vi "LaserMaster.vi"() -> ()   [LabVIEW 2014]
uses:
  <vilib>/Instr/_visa.llb/VISA Configure Serial Port (Instr).vi
  <vilib>/Utility/file.llb/Write To Spreadsheet File (string).vi
panel:
  out "Humidity Threshold":dbl
  in  "Power (mW) 2":dbl format="%#.0f"
  out "SavePath":path
  out "Start time":timestamp
  out "Step":dbl
  out "State next step":string
  in  "stop":bool
  out "Query backup List":string[][](array[string])=[["?L", " 0\r"], ["?K", " 0\r"], ["?F", " 0\r"], ["?FH", " 2\r"], ["?SHUTTER", " 0\r"], ["?UF", " 0\r"], ["?PHLDC", " 1\r"], ["?PZTMC", " 0\r"], ["?PZTXC", " 2.24\r"], ["?PZTYC", " 2.14\r"], ["?PHLDP", " 0\r"], ["?PZTMP", " 0\r"], ["?PZTXP", " 2.58\r"], ["?PXTYP", "  Query Error:?PXTYP\r"], ["?PTRK", "  Query Error:?PTRK\r"], ["?MDLK", " 0\r"], ["?PP", " 0.80\r"], ["?TS", " 0\r"], ["?SM", " 1\r"], ["?HM", " 1\r"], ["?VW", " 850\r"], ["?STPRPOS", " 2096\r"], ["?C", " 0.00\r"], ["?D1C", " 0.08\r"], ["?D2C", " -0.43\r"], ["?BT", " 20.07\r"], ["?D1T", " 24.20\r"], ["?D2T", " 24.20\r"], ["?VT", " 20.72\r"], ["?LBOT", " 148.45\r"], ["?ET", " 39.01\r"], ["?D1ST", " 24.20\r"], ["?D2ST", " 24.20\r"], ["?VST", " 30.00\r"], ["?LBOST", " 148.41\r"], ["?EST", " 39.00\r"], ["?D1TD", " 500.12\r"], ["?D2TD", " 464.53\r"], ["?VD", " 0.00\r"], ["?LBOD", " 5358.08\r"], ["?ED", " 2152.46\r"], ["?D1HST", " 21.35\r"], ["?D2HST", " 21.48\r"], ["?LBOH", " 1\r"], ["?LRS", " 2\r"], ["?D1SS", " 1\r"], ["?D2SS", " 1\r"], ["?VSS", " 0\r"], ["?LBOSS", " 1\r"], ["?ESS", " 1\r"], ["?D1H", "  351.54\r"], ["?D2H", "  351.52\r"], ["?HH", " 37\r"], ["?D1V", " 0.19\r"], ["?D2V", " 0.18\r"], ["?SV", " 8.26,8.26,9.57\r"], ["?MB", "  Query Error:?MB\r"], ["?PI", " 2BC\r"], ["?BV", " 13.24\r"], ["?AMDLK", " 1\r"], ["?PZTS", "  Query Error:?PZTS\r"], ["?TMAX", " 1080\r"], ["?TMIN", " 680\r"], ["?ALIGN", " 0\r"], ["?ALIGNP", " 250\r"], ["?ALIGNW", " 730\r"], ["?LFP", " 0\r"], ["?PZTXCM", " 8.11\r"], ["?PZTXCP", " -10.30\r"], ["?PZTXPM", " 8.11\r"], ["?PZTXPP", " 3.06\r"], ["?PZTYCM", " 8.11\r"], ["?PZTYCP", " -14.28\r"], ["?PZTYPM", " 8.11\r"], ["?PZTYPP", " 11.74\r"], ["?RH", " 0\r"], ["?SN", " 9571\r"], ["?ST", " Standby\r"], ["?GDDCURVE", " 0\r"], ["?GDD", " 0\r"], ["?GDDCURVEN", " ZERO\r"], ["?CURVEN", " OUT OF RANGE\r"], ["?COMP", " 1\r"], ["?HMCOMP", " 1\r"], ["?GDDMAX", " 17333\r"], ["?GDDMIN", "0"]]
  out "Laser Info":i32
  out "Shutter off time":dbl
  out "Quiting":dbl
  out "Backuper state":string
  in  "Tab Control":T1(tab)
  in  "Auto":bool
  out "Baseplate Temp (C)":dbl(slide) scale=20.0..40.0
  in  "Dither hold":bool
  in  "Shutter":bool
  in  "Lock":bool
  out "Laser Status":bool
  out "Power (mW)":dbl(knob) scale=0.0..5000.0
  out "Walking":bool
  out "Sleeping":bool
  out "ModeLocked":bool
  out "Backing up":bool
  in  "Wavelength":dbl
  in  "GDD":dbl
  in  "Align":bool
  in  "QUIT":bool
  out "Max":string
  in  "Dither auto":dbl=120.0
  in  "Dither timer":dbl=5.0
  out "Faults":string
  in  "Home motor":bool
  in  "Optimize":bool
  in  "WV Walk":bool
  in  "Auto-Standby\nTime (min)":dbl=120.0
  in  "Sleep":bool
  in  "Backup":bool
  in  "Auto-Backup \nIdle Time (min)":dbl=30.0
  out "Operating Status":string
  out "Tunning Status":i32
  out "Idle Time":dbl format="%.1f"
  out "Laser On Time":dbl format="%#.1f"
  in  "Laser Control":bool
  in  "Command Line":string
  out "Laser Response":string
  in  "Refresh":bool
  out "Query List":string[][](array[string])
  out "queue #":i32
  # "LASER"
  # "LASER fine-tune"
  # "BACKUP"
  # "Timers"
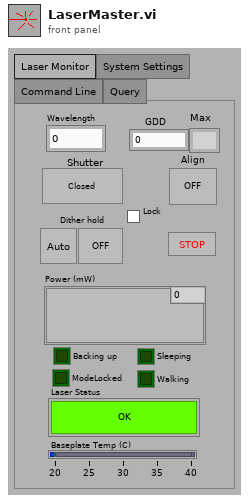
[diagram p1: front panel]
types:
  T1 = enum32{"Laser Monitor", "System Settings", "Command Line", "Query"}
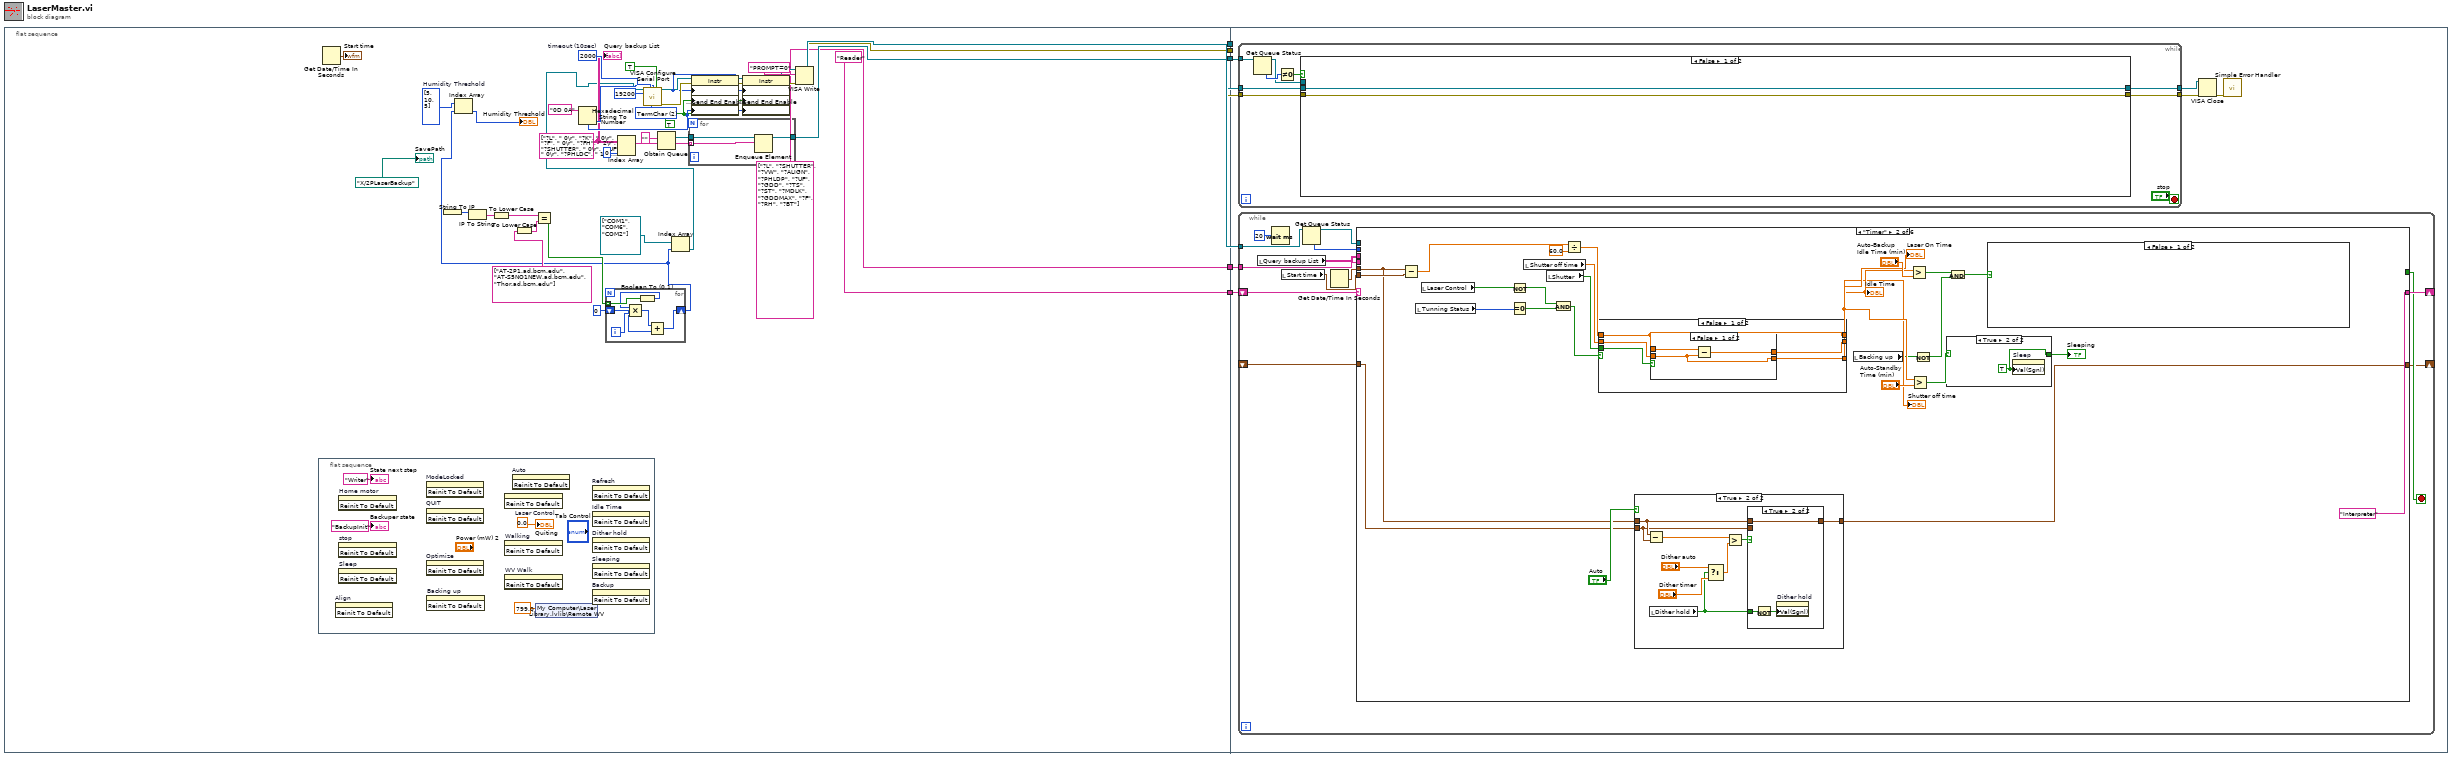
[diagram p0: block diagram]
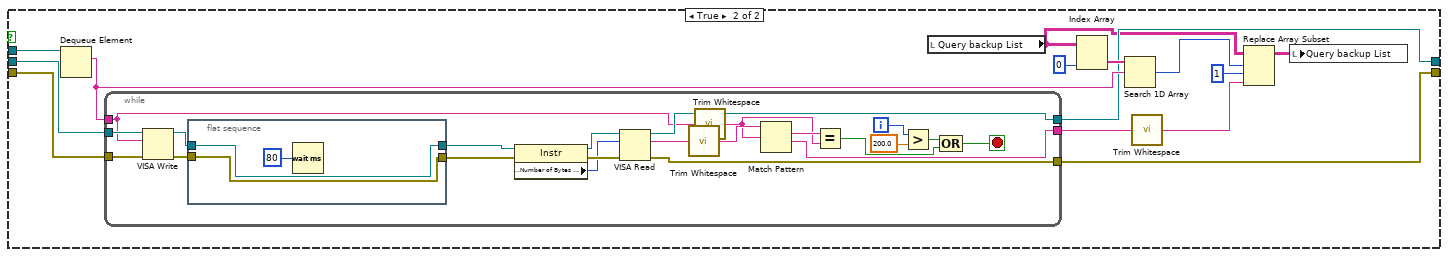
[diagram p2: hidden frame]
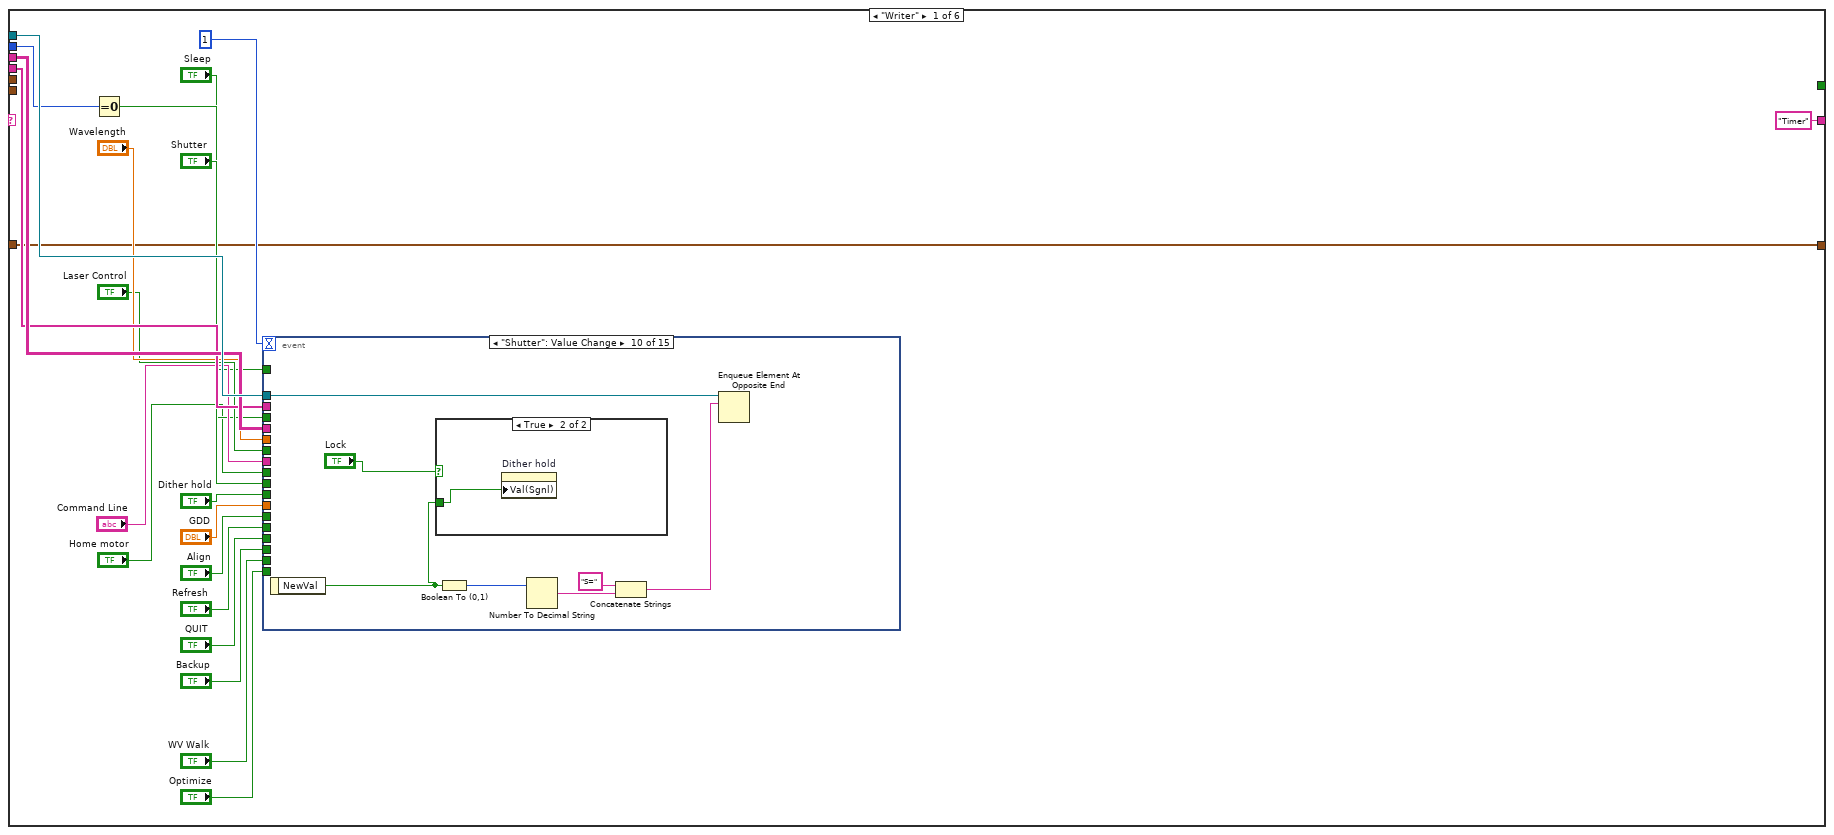
[diagram p3: hidden frame]
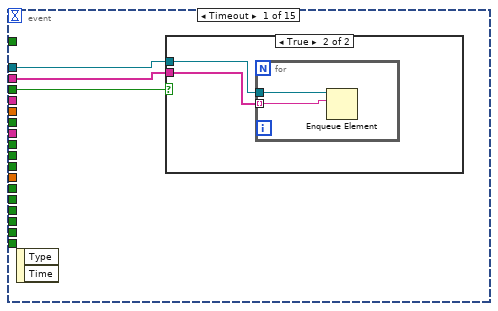
[diagram p4: hidden frame]
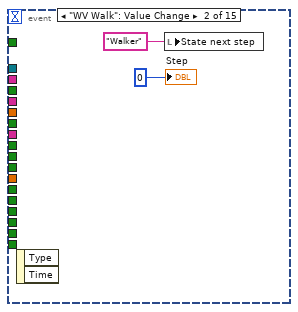
[diagram p6: hidden frame]
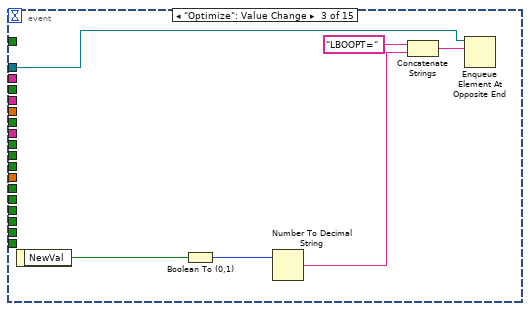
[diagram p7: hidden frame]
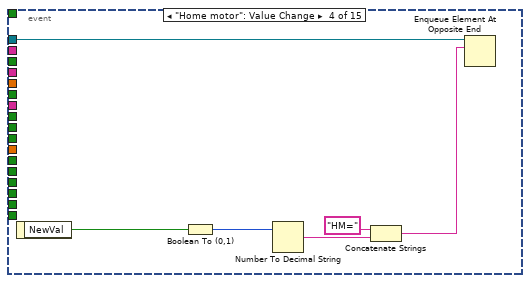
[diagram p8: hidden frame]
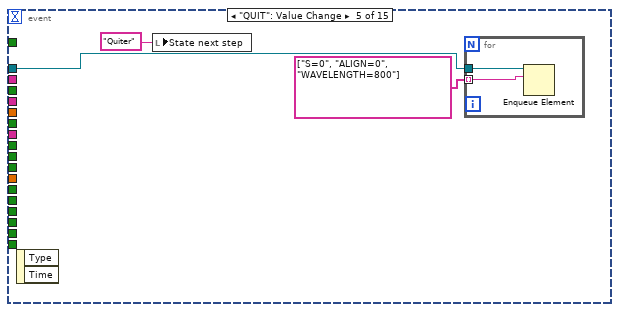
[diagram p9: hidden frame]
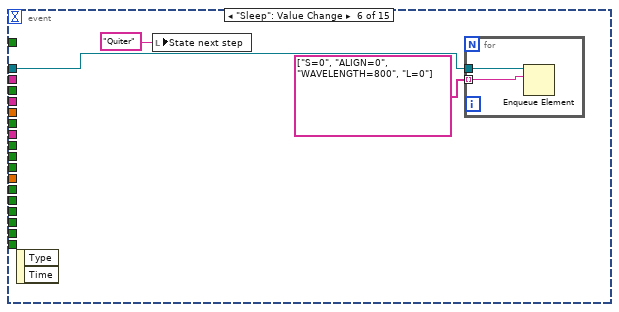
[diagram p10: hidden frame]
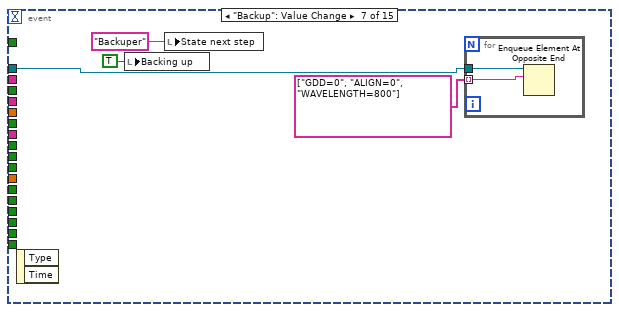
[diagram p11: hidden frame]
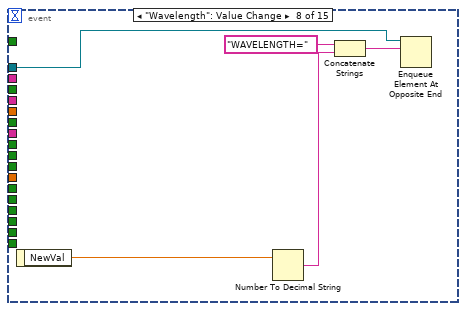
[diagram p12: hidden frame]
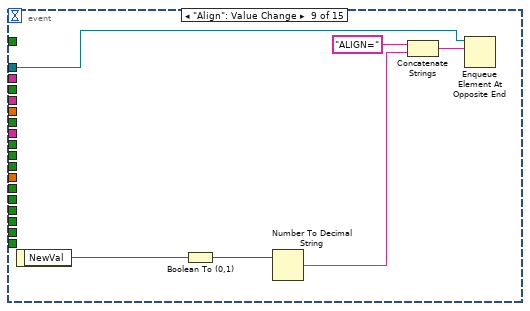
[diagram p13: hidden frame]
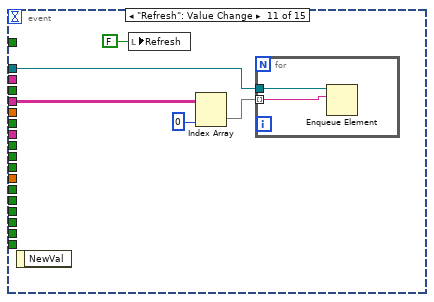
[diagram p15: hidden frame]
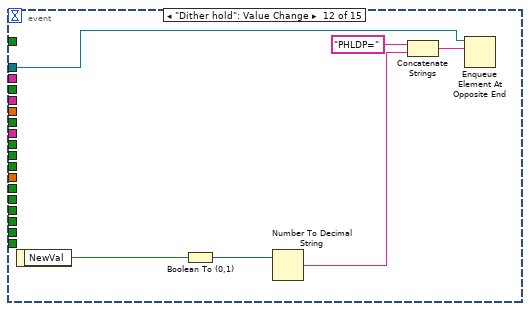
[diagram p16: hidden frame]
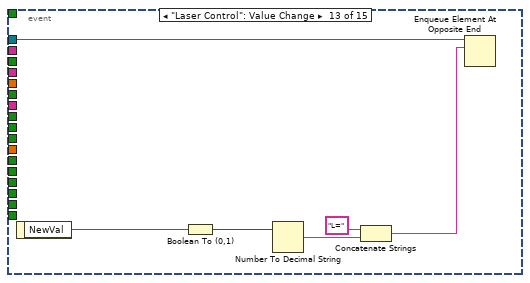
[diagram p17: hidden frame]
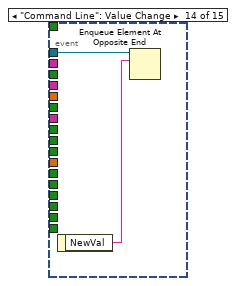
[diagram p18: hidden frame]
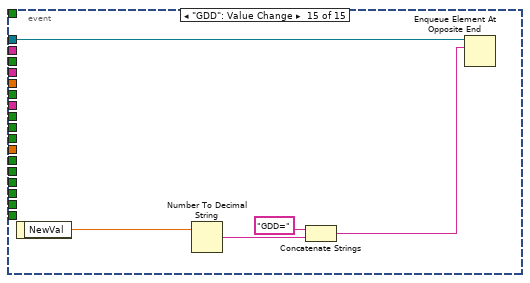
[diagram p19: hidden frame]
diagram:
  n1 = flat-sequence {
    tunnel: [w32] -> w5
    tunnel: [w31] -> w4
    tunnel: [w22] -> w3
    tunnel: [string[] ["?L", "?SHUTTER", "?VW", "?ALIGN", "?PHLDP", "?UF", "?GDD", "?TS", "?ST", "?MDLK", "?GDDMAX", "?F", "?RH", "?BT"]] -> w2
    tunnel: ["Reader"] -> w1
    tunnel: w5 -> [w60]
    tunnel: w4 -> [w57]
    tunnel: w3 -> [w61]
    tunnel: w2 -> [w63]
    tunnel: w1 -> [w62]
    frame #0 {
      w8 = i32[] [5, 10, 5]  # Humidity Threshold
      w21 = string[][] [["?L", " 0\r"], ["?K", " 0\r"], ["?F", " 0\r"], ["?FH", " 2\r"], ["?SHUTTER", " 0\r"], ["?UF", " 0\r"], ["?PHLDC", " 1\r"], ["?PZTMC", " 0\r"], ["?PZTXC", " 2.24\r"], ["?PZTYC", " 2.14\r"], ["?PHLDP", " 0\r"], ["?PZTMP", " 0\r"], ["?PZTXP", " 2.58\r"], ["?PXTYP", "  Query Error:?PXTYP\r"], ["?PTRK", "  Query Error:?PTRK\r"], ["?MDLK", " 0\r"], ["?PP", " 0.80\r"], ["?TS", " 0\r"], ["?SM", " 1\r"], ["?HM", " 1\r"], ["?VW", " 850\r"], ["?STPRPOS", " 2096\r"], ["?C", " 0.00\r"], ["?D1C", " 0.08\r"], ["?D2C", " -0.43\r"], ["?BT", " 20.07\r"], ["?D1T", " 24.20\r"], ["?D2T", " 24.20\r"], ["?VT", " 20.72\r"], ["?LBOT", " 148.45\r"], ["?ET", " 39.01\r"], ["?D1ST", " 24.20\r"], ["?D2ST", " 24.20\r"], ["?VST", " 30.00\r"], ["?LBOST", " 148.41\r"], ["?EST", " 39.00\r"], ["?D1TD", " 500.12\r"], ["?D2TD", " 464.53\r"], ["?VD", " 0.00\r"], ["?LBOD", " 5358.08\r"], ["?ED", " 2152.46\r"], ["?D1HST", " 21.35\r"], ["?D2HST", " 21.48\r"], ["?LBOH", " 1\r"], ["?LRS", " 2\r"], ["?D1SS", " 1\r"], ["?D2SS", " 1\r"], ["?VSS", " 0\r"], ["?LBOSS", " 1\r"], ["?ESS", " 1\r"], ["?D1H", "  351.54\r"], ["?D2H", "  351.52\r"], ["?HH", " 37\r"], ["?D1V", " 0.19\r"], ["?D2V", " 0.18\r"], ["?SV", " 8.26,8.26,9.57\r"], ["?MB", "  Query Error:?MB\r"], ["?PI", " 2BC\r"], ["?BV", " 13.24\r"], ["?AMDLK", " 1\r"], ["?PZTS", "  Query Error:?PZTS\r"], ["?TMAX", " 1080\r"], ["?TMIN", " 680\r"], ["?ALIGN", " 0\r"], ["?ALIGNP", " 250\r"], ["?ALIGNW", " 730\r"], ["?LFP", " 0\r"], ["?PZTXCM", " 8.11\r"], ["?PZTXCP", " -10.30\r"], ["?PZTXPM", " 8.11\r"], ["?PZTXPP", " 3.06\r"], ["?PZTYCM", " 8.11\r"], ["?PZTYCP", " -14.28\r"], ["?PZTYPM", " 8.11\r"], ["?PZTYPP", " 11.74\r"], ["?RH", " 0\r"], ["?SN", " 9571\r"], ["?ST", " Standby\r"], ["?GDDCURVE", " 0\r"], ["?GDD", " 0\r"], ["?GDDCURVEN", " ZERO\r"], ["?CURVEN", " OUT OF RANGE\r"], ["?COMP", " 1\r"], ["?HMCOMP", " 1\r"], ["?GDDMAX", " 17333\r"], ["?GDDMIN", "0"]] ("Query backup List")
      w35 = TRUE ("Message Based Settings:Send End Enable")
      w36 = u16 2 items=["None", "LastBit", "TermChar", "Break"] ("Serial Settings:Serial End Mode for Writes")
      w43 = u32 2000  # timeout (10sec)
      n2 = flat-sequence {
        frame #0 {
          n3 = invoke on="Align" class="Bool (strict)" method="Reinit To Default"() -> ()  [unwired: 3 in, 3 out]
          n4 = invoke on="Home motor" class="Bool" method="Reinit To Default"() -> ()  [unwired: 3 in, 3 out]
          n5 = invoke on="stop" class="Bool (strict)" method="Reinit To Default"() -> ()  [unwired: 3 in, 3 out]
          n6 = invoke on="Sleep" class="Bool (strict)" method="Reinit To Default"() -> ()  [unwired: 3 in, 3 out]
          n7 = invoke on="ModeLocked" class="Bool (strict)" method="Reinit To Default"() -> ()  [unwired: 3 in, 3 out]
          n8 = invoke on="QUIT" class="Bool (strict)" method="Reinit To Default"() -> ()  [unwired: 3 in, 3 out]
          n9 = invoke on="Optimize" class="Bool" method="Reinit To Default"() -> ()  [unwired: 3 in, 3 out]
          n10 = invoke on="Backing up" class="Bool (strict)" method="Reinit To Default"() -> ()  [unwired: 3 in, 3 out]
          n11 = invoke on="Laser Control" class="Bool (strict)" method="Reinit To Default"() -> ()  [unwired: 3 in, 3 out]
          n12 = invoke on="Walking" class="Bool (strict)" method="Reinit To Default"() -> ()  [unwired: 3 in, 3 out]
          n13 = invoke on="WV Walk" class="Bool (strict)" method="Reinit To Default"() -> ()  [unwired: 3 in, 3 out]
          n14 = invoke on="Auto" class="Bool (strict)" method="Reinit To Default"() -> ()  [unwired: 3 in, 3 out]
          n15 = shared-variable "My Computer\\Laser Library.lvlib\\Remote WV"(799.0 ("Remote WV")) -> ()  [unwired: 1 in, 1 out]
          n16 = invoke on="Refresh" class="Bool (strict)" method="Reinit To Default"() -> ()  [unwired: 3 in, 3 out]
          n17 = invoke on="Idle Time" class="DigNum (strict)" method="Reinit To Default"() -> ()  [unwired: 3 in, 3 out]
          n18 = invoke on="Dither hold" class="Bool (strict)" method="Reinit To Default"() -> ()  [unwired: 3 in, 3 out]
          n19 = invoke on="Sleeping" class="Bool (strict)" method="Reinit To Default"() -> ()  [unwired: 3 in, 3 out]
          n20 = invoke on="Backup" class="Bool (strict)" method="Reinit To Default"() -> ()  [unwired: 3 in, 3 out]
          "Backuper state" <- "BackupInit"
          "Quiting" <- 0.0 ("Quiting")
          "State next step" <- "Writer"
        }
      }
      n21 = Get Date/Time In Seconds() -> (seconds since 1Jan1904=→"Start time":timestamp)
      n22 = String To IP() -> (0:w17:u32)  [unwired: 1 in]
      n23 = IP To String(2:w17) -> (0:w14:string)  [unwired: 1 in]
      n24 = To Lower Case(string=w14) -> (all lower case string=w16:string)
      n25 = To Lower Case(string=string[] ["AT-2P1.ad.bcm.edu", "AT-S5NO1NEW.ad.bcm.edu", "Thor.ad.bcm.edu"]) -> (all lower case string=w15:string[])
      n26 = Equal?(x=w16, y=w15) -> (x = y?=w11:bool[])
      n27 = Hexadecimal String To Number(string="0D 0A") -> (number=w34:u32)  [unwired: 2 in, 1 out]
      n28 = for {
        tunnel: w11 -> [w48] mode=indexing
        shift-right: [w44] -> w7
        shift-left: 0 -> [w45]
        i -> [w49]
        n29 = Boolean To (0,1)(Boolean=w48) -> (0, 1=w47:i16)
        n30 = Multiply(x=w47, y=w49) -> (x*y=w46:i32)
        n31 = Add(x=w46, y=w45) -> (x+y=w44:i32)
      }
      n32 = Index Array(array=w8, index=w7) -> (element=→"Humidity Threshold":i32)
      n33 = Index Array(array=w21, index (col)=0 ("disabled index (col)")) -> (element=w24:string[])  [unwired: 1 in]
      n34 = Obtain Queue(element data type="") -> (queue out=w26:refnum<queue>)  [unwired: 4 in, 2 out]
      n35 = Index Array(array=refnum<visa-resource-name>[] ["COM1", "COM6", "COM2"], index=w7) -> (element=w9:refnum<visa-resource-name>)
      n36 = call-poly "VISA Configure Serial Port"("VISA resource name"=w9, "timeout (10sec)"=w43, "termination char\n(0xA = '\\n' = LF)"=w34, "Enable Termination\nChar (T)"=TRUE ("Enable Termination\nChar (T)"), "baud rate (9600)"=u32 19200) -> ("VISA resource name out"=w40:refnum<visa-resource-name>, "error out"=w39:errorcluster)  [unwired: 5 in, 4 out]
      n37 = for {
        tunnel: w26 -> [w56]
        tunnel: w24 -> [w55] mode=indexing
        tunnel: [w54] -> w22
        n38 = Enqueue Element(queue=w56, element=w55) -> (queue out=w54:refnum<queue>)  [unwired: 2 in, 2 out]
      }
      n39 = property class="Instr"(reference=w40, error in=w39, "Serial Settings:End Mode for Writes"=w36, "Message Based Settings:Send End Enable"=w35, "Message Based Settings:Termination Character"=w34) -> (reference out=w38:refnum<visa-resource-name>, error out=w37:errorcluster)
      n40 = property class="Instr"(reference=w38, error in=w37, "Serial Settings:End Mode for Writes"=w36, "Message Based Settings:Send End Enable"=w35, "Message Based Settings:Termination Character"=w34) -> (reference out=w29:refnum<visa-resource-name>, error out=w28:errorcluster)
      n41 = VISA Write(VISA resource name=w29, write buffer="PROMPT=0", error in (no error)=w28) -> (VISA resource name out=w32:refnum<visa-resource-name>, error out=w31:errorcluster)  [unwired: 1 out]
      "Query backup List" <- w21
      "SavePath" <- path "X:/2PLaserBackup"
    }
    frame #1 {
      n42 = while {
        tunnel: w61 -> [w68]
        tunnel: w60 -> [w73]
        tunnel: [w72] -> w59
        tunnel: [w71] -> w58
        tunnel: w57 -> [w70]
        stop <- "stop" stop-if-true
        n43 = Get Queue Status(queue=w68) -> (queue out=w65:refnum<queue>, # elements in queue=w67:i32)  [unwired: 2 in, 6 out]
        n44 = Not Equal To 0?(x=w67) -> (x != 0?=w66:bool)
        n45 = case shown="False" w66 {
          tunnel: w65 -> [_ w82]
          tunnel: w73 -> [w75 w81]
          tunnel: [w75 w80] -> w72
          tunnel: [w74 w79] -> w71
          tunnel: w70 -> [w74 w78]
          frame False {
          }
          frame True {
            n46 = Dequeue Element(queue=w82) -> (element=w84:string)  [unwired: 2 in, 3 out]
            n47 = while {
              tunnel: w81 -> [w111]
              tunnel: w78 -> [w110]
              tunnel: [w109] -> w80
              tunnel: [w108] -> w79
              tunnel: w84 -> [w96]
              tunnel: [w104] -> w85
              i -> [w94]
              stop <- w91 stop-if-true
              n48 = VISA Write(VISA resource name=w111, write buffer=w96, error in (no error)=w110) -> (VISA resource name out=w102:refnum<visa-resource-name>, error out=w99:errorcluster)  [unwired: 1 out]
              n49 = flat-sequence {
                tunnel: [w114] -> w101
                tunnel: w102 -> [w114]
                tunnel: w99 -> [w113]
                tunnel: [w113] -> w100
                frame #0 {
                  n50 = Wait (ms)(milliseconds to wait=u32 80) -> ()  [unwired: 1 out]
                }
              }
              n51 = property class="Instr"(reference=w101, error in=w100) -> (reference out=w107:refnum<visa-resource-name>, error out=w106:errorcluster, "Serial Settings:Number of Bytes at Serial Port"=w105:u32)
              n52 = VISA Read(VISA resource name=w107, byte count=w105, error in (no error)=w106) -> (VISA resource name out=w109:refnum<visa-resource-name>, read buffer=w98:string, error out=w108:errorcluster)  [unwired: 1 out]
              n53 = call <vilib>:"Trim Whitespace.vi"("string"=w98) -> ("trimmed string"=w97:string)  [unwired: 1 in]
              n54 = call <vilib>:"Trim Whitespace.vi"("string"=w96) -> ("trimmed string"=w90:string)  [unwired: 1 in]
              n55 = Match Pattern(string=w97, regular expression=w90) -> (match substring=w103:string, after substring=w104:string)  [unwired: 1 in, 2 out]
              n56 = Equal?(x=w103, y=w90) -> (x = y?=w92:bool)
              n57 = Greater?(x=w94, y=200.0) -> (0:w93:bool)
              n58 = Compound Arithmetic op=OR(w93, w92) -> (w91:bool)
            }
            n59 = local read "Query backup List"() -> (w77:string[][])
            n60 = Index Array(array=w77, index (col)=0 ("index (row)")) -> (element=w88:string[])  [unwired: 1 in]
            n61 = Search 1D Array(1D array=w88, element=w84) -> (index of element=w86:i32)  [unwired: 1 in]
            n62 = call <vilib>:"Trim Whitespace.vi"("string"=w85) -> ("trimmed string"=w83:string)  [unwired: 1 in]
            n63 = Replace Array Subset(array=w77, new element=w83, index (row)=w86, index (col)=1 ("disabled index (col)")) -> (w76:string[][])
            n64 = local write "Query backup List"(w76) -> ()
          }
        }
      }
      n65 = while {
        tunnel: w61 -> [w124]
        tunnel: w63 -> [w125]
        shift-right: [w126] -> _
        shift-left: w62 -> [w127]
        shift-right: [w116] -> _
        shift-left: _ -> [w115]
        stop <- w121 stop-if-true
        n66 = local read "Query backup List"() -> (w123:string[][])
        n67 = Wait (ms)(milliseconds to wait=u32 20) -> ()  [unwired: 1 out]
        n68 = local read "Start time"() -> (w117:timestamp)
        n69 = Get Queue Status(queue=w124) -> (queue out=w120:refnum<queue>, # elements in queue=w119:i32)  [unwired: 2 in, 6 out]
        n70 = Get Date/Time In Seconds() -> (seconds since 1Jan1904=w118:timestamp)
        n71 = case shown="\"Timer\"" w127 {
          tunnel: w120 -> [w149 _ _ _ _ _]
          tunnel: w123 -> [w148 _ w302 _ w457 _]
          tunnel: w125 -> [w147 _ w303 _ _ _]
          tunnel: ["Timer" "Interpreter" w301 "Writer" "Writer" w483] -> w126
          tunnel: w119 -> [w146 _ w300 _ _ w485]
          tunnel: [_ _ _ _ _ w482] -> w121
          tunnel: w118 -> [_ w233 _ _ _ _]
          tunnel: w117 -> [_ w237 _ _ _ _]
          tunnel: [w128 w234 w299 w439 w454 w481] -> w116
          tunnel: w115 -> [w128 w232 w299 w439 w454 w481]
          frame "Writer" {
            n72 = Equal To 0?(x=w146) -> (x = 0?=w134:bool)
            n73 = event shown="[9] \"Shutter\": Value Change" {
              selector: _ -> [_ _ _ _ _ _ _ _ _ _ _ _ _ _ _]
              dyn-events: _ -> [_ _ _ _ _ _ _ _ _ _ _ _ _ _ _]
              timeout: 1 -> [_ _ _ _ _ _ _ _ _ _ _ _ _ _ _]
              tunnel: w149 -> [w152 _ w159 w166 w172 w176 w183 w188 w193 w200 w207 w214 w219 w226 w228]
              tunnel: "Shutter" -> [_ _ _ _ _ _ _ _ _ _ _ _ _ _ _]
              tunnel: "Dither hold" -> [_ _ _ _ _ _ _ _ _ _ _ _ _ _ _]
              tunnel: "GDD" -> [_ _ _ _ _ _ _ _ _ _ _ _ _ _ _]
              tunnel: "Align" -> [_ _ _ _ _ _ _ _ _ _ _ _ _ _ _]
              tunnel: "Wavelength" -> [_ _ _ _ _ _ _ _ _ _ _ _ _ _ _]
              tunnel: "Laser Control" -> [_ _ _ _ _ _ _ _ _ _ _ _ _ _ _]
              tunnel: "Command Line" -> [_ _ _ _ _ _ _ _ _ _ _ _ _ _ _]
              tunnel: w148 -> [_ _ _ _ _ _ _ _ _ _ w206 _ _ _ _]
              tunnel: "Refresh" -> [_ _ _ _ _ _ _ _ _ _ _ _ _ _ _]
              tunnel: w147 -> [w151 _ _ _ _ _ _ _ _ _ _ _ _ _ _]
              tunnel: "QUIT" -> [_ _ _ _ _ _ _ _ _ _ _ _ _ _ _]
              tunnel: "Backup" -> [_ _ _ _ _ _ _ _ _ _ _ _ _ _ _]
              tunnel: w134 -> [w150 _ _ _ _ _ _ _ _ _ _ _ _ _ _]
              tunnel: "WV Walk" -> [_ _ _ _ _ _ _ _ _ _ _ _ _ _ _]
              tunnel: "Optimize" -> [_ _ _ _ _ _ _ _ _ _ _ _ _ _ _]
              tunnel: "Home motor" -> [_ _ _ _ _ _ _ _ _ _ _ _ _ _ _]
              tunnel: "Sleep" -> [_ _ _ _ _ _ _ _ _ _ _ _ _ _ _]
              event Timeout {
                n74 = event-data() -> ()  [unwired: 1 in, 2 out]
                n75 = case shown="True" w150 {
                  tunnel: w152 -> [_ w154]
                  tunnel: w151 -> [_ w153]
                  frame False {
                  }
                  frame True {
                    n76 = for {
                      tunnel: w154 -> [w156]
                      tunnel: w153 -> [w155] mode=indexing
                      n77 = Enqueue Element(queue=w156, element=w155) -> ()  [unwired: 2 in, 3 out]
                    }
                  }
                }
              }
              event "WV Walk": Value Change {
                n78 = event-data() -> ()  [unwired: 1 in, 2 out]
                n79 = local write "State next step"("Walker") -> ()
                "Step" <- 0
              }
              event "Optimize": Value Change {
                n80 = event-data() -> ("NewVal"=w160:bool)  [unwired: 1 in]
                n81 = Boolean To (0,1)(Boolean=w160) -> (0, 1=w163:i16)
                n82 = Number To Decimal String(number=w163) -> (decimal integer string=w164:string)  [unwired: 1 in]
                n83 = Concatenate Strings("LBOOPT=", w164) -> (w161:string)
                n84 = Enqueue Element At Opposite End(queue=w159, element=w161) -> ()  [unwired: 2 in, 3 out]
              }
              event "Home motor": Value Change {
                n85 = event-data() -> ("NewVal"=w165:bool)  [unwired: 1 in]
                n86 = Boolean To (0,1)(Boolean=w165) -> (0, 1=w169:i16)
                n87 = Number To Decimal String(number=w169) -> (decimal integer string=w170:string)  [unwired: 1 in]
                n88 = Concatenate Strings("HM=", w170) -> (w167:string)
                n89 = Enqueue Element At Opposite End(queue=w166, element=w167) -> ()  [unwired: 2 in, 3 out]
              }
              event "QUIT": Value Change {
                n90 = event-data() -> ()  [unwired: 1 in, 2 out]
                n91 = local write "State next step"("Quiter") -> ()
                n92 = for {
                  tunnel: w172 -> [w175]
                  tunnel: string[] ["S=0", "ALIGN=0", "WAVELENGTH=800"] -> [w174] mode=indexing
                  n93 = Enqueue Element(queue=w175, element=w174) -> ()  [unwired: 2 in, 3 out]
                }
              }
              event "Sleep": Value Change {
                n94 = event-data() -> ()  [unwired: 1 in, 2 out]
                n95 = local write "State next step"("Quiter") -> ()
                n96 = for {
                  tunnel: w176 -> [w180]
                  tunnel: string[] ["S=0", "ALIGN=0", "WAVELENGTH=800", "L=0"] -> [w179] mode=indexing
                  n97 = Enqueue Element(queue=w180, element=w179) -> ()  [unwired: 2 in, 3 out]
                }
              }
              event "Backup": Value Change {
                n98 = event-data() -> ()  [unwired: 1 in, 2 out]
                n99 = local write "Backing up"(TRUE ("Backing up ...")) -> ()
                n100 = local write "State next step"("Backuper") -> ()
                n101 = for {
                  tunnel: string[] ["GDD=0", "ALIGN=0", "WAVELENGTH=800"] -> [w186] mode=indexing
                  tunnel: w183 -> [w185]
                  n102 = Enqueue Element At Opposite End(queue=w185, element=w186) -> ()  [unwired: 2 in, 3 out]
                }
              }
              event "Wavelength": Value Change {
                n103 = event-data() -> ("NewVal"=w187:dbl)  [unwired: 1 in]
                n104 = Number To Decimal String(number=w187) -> (decimal integer string=w190:string)  [unwired: 1 in]
                n105 = Concatenate Strings("WAVELENGTH=", w190) -> (w191:string)
                n106 = Enqueue Element At Opposite End(queue=w188, element=w191) -> ()  [unwired: 2 in, 3 out]
              }
              event "Align": Value Change {
                n107 = event-data() -> ("NewVal"=w192:bool)  [unwired: 1 in]
                n108 = Boolean To (0,1)(Boolean=w192) -> (0, 1=w196:i16)
                n109 = Number To Decimal String(number=w196) -> (decimal integer string=w197:string)  [unwired: 1 in]
                n110 = Concatenate Strings("ALIGN=", w197) -> (w194:string)
                n111 = Enqueue Element At Opposite End(queue=w193, element=w194) -> ()  [unwired: 2 in, 3 out]
              }
              event "Shutter": Value Change {
                n112 = event-data() -> ("NewVal"=w198:bool)  [unwired: 1 in]
                n113 = case shown="True" "Lock" {
                  tunnel: w198 -> [_ w205]
                  frame False {
                  }
                  frame True {
                    n114 = property on="Dither hold" class="Bool (strict)"("Val(Sgnl)"=w205) -> ()  [unwired: 2 in, 2 out]
                  }
                }
                n115 = Boolean To (0,1)(Boolean=w198) -> (0, 1=w203:i16)
                n116 = Number To Decimal String(number=w203) -> (decimal integer string=w204:string)  [unwired: 1 in]
                n117 = Concatenate Strings("S=", w204) -> (w201:string)
                n118 = Enqueue Element At Opposite End(queue=w200, element=w201) -> ()  [unwired: 2 in, 3 out]
              }
              event "Refresh": Value Change {
                n119 = event-data() -> ()  [unwired: 1 in, 1 out]
                n120 = local write "Refresh"(FALSE ("Backup")) -> ()
                n121 = Index Array(array=w206, index (col)=0 ("disabled index (col)")) -> (element=w209:string[])  [unwired: 1 in]
                n122 = for {
                  tunnel: w207 -> [w212]
                  tunnel: w209 -> [w211] mode=indexing
                  n123 = Enqueue Element(queue=w212, element=w211) -> ()  [unwired: 2 in, 3 out]
                }
              }
              event "Dither hold": Value Change {
                n124 = event-data() -> ("NewVal"=w213:bool)  [unwired: 1 in]
                n125 = Boolean To (0,1)(Boolean=w213) -> (0, 1=w217:i16)
                n126 = Number To Decimal String(number=w217) -> (decimal integer string=w218:string)  [unwired: 1 in]
                n127 = Concatenate Strings("PHLDP=", w218) -> (w215:string)
                n128 = Enqueue Element At Opposite End(queue=w214, element=w215) -> ()  [unwired: 2 in, 3 out]
              }
              event "Laser Control": Value Change {
                n129 = event-data() -> ("NewVal"=w220:bool)  [unwired: 1 in]
                n130 = Boolean To (0,1)(Boolean=w220) -> (0, 1=w223:i16)
                n131 = Number To Decimal String(number=w223) -> (decimal integer string=w224:string)  [unwired: 1 in]
                n132 = Concatenate Strings("L=", w224) -> (w221:string)
                n133 = Enqueue Element At Opposite End(queue=w219, element=w221) -> ()  [unwired: 2 in, 3 out]
              }
              event "Command Line": Value Change {
                n134 = event-data() -> ("NewVal"=w225:string)  [unwired: 1 in]
                n135 = Enqueue Element At Opposite End(queue=w226, element=w225) -> ()  [unwired: 2 in, 3 out]
              }
              event "GDD": Value Change {
                n136 = event-data() -> ("NewVal"=w227:dbl)  [unwired: 1 in]
                n137 = Number To Decimal String(number=w227) -> (decimal integer string=w230:string)  [unwired: 1 in]
                n138 = Concatenate Strings("GDD=", w230) -> (w231:string)
                n139 = Enqueue Element At Opposite End(queue=w228, element=w231) -> ()  [unwired: 2 in, 3 out]
              }
            }
          }
          frame "Timer" {
            n140 = Subtract(x=w233, y=w237) -> (x-y=w240:dbl)
            n141 = local read "Tunning Status"() -> (w257:i32)
            n142 = local read "Laser Control"() -> (w256:bool)
            n143 = Not(x=w256) -> (.not. x?=w252:bool)
            n144 = Equal To 0?(x=w257) -> (x = 0?=w251:bool)
            n145 = local read "Shutter off time"() -> (w247:dbl)
            n146 = local read "Shutter"() -> (w248:bool)
            n147 = And(x=w252, y=w251) -> (x .and. y?=w253:bool)
            n148 = Divide(x=w240, y=60.0 ("x")) -> (x/y=w238:dbl)
            n149 = case shown="False" w253 {
              tunnel: [w273 w284] -> w250
              tunnel: [w277 w284] -> w249
              tunnel: w248 -> [w276 _]
              tunnel: w247 -> [w275 _]
              tunnel: [w274 w284] -> w246
              tunnel: w238 -> [w273 _]
              frame False {
                n150 = case shown="False" w276 {
                  tunnel: [w280 0] -> w277
                  tunnel: w273 -> [w279 w281]
                  tunnel: w275 -> [w278 _]
                  tunnel: [w278 w281] -> w274
                  frame False {
                    n151 = Subtract(x=w279, y=w278) -> (x-y=w280:dbl)
                  }
                  frame True {
                  }
                }
              }
              frame True {
                w284 = 0
                n152 = Get Date/Time In Seconds() -> (seconds since 1Jan1904=w283:timestamp)
                n153 = local write "Start time"(w283) -> ()
              }
            }
            "Laser On Time" <- w250
            "Idle Time" <- w249
            "Shutter off time" <- w246
            n154 = case shown="True" "Auto" {
              tunnel: w233 -> [w259 w266]
              tunnel: [w259 w265] -> w234
              tunnel: w232 -> [_ w264]
              frame False {
              }
              frame True {
                n155 = Subtract(x=w266, y=w264) -> (x-y=w268:dbl)
                n156 = local read "Dither hold"() -> (w260:bool)
                n157 = Select(t="Dither auto", s=w260, f="Dither timer") -> (s? t:f=w261:dbl)
                n158 = Greater?(x=w268, y=w261) -> (0:w267:bool)
                n159 = case shown="True" w267 {
                  tunnel: w266 -> [_ w272]
                  tunnel: [w269 w272] -> w265
                  tunnel: w264 -> [w269 _]
                  tunnel: w260 -> [_ w271]
                  frame False {
                  }
                  frame True {
                    n160 = Not(x=w271) -> (.not. x?=w270:bool)
                    n161 = property on="Dither hold" class="Bool (strict)"("Val(Sgnl)"=w270) -> ()  [unwired: 2 in, 2 out]
                  }
                }
              }
            }
            n162 = local read "Backing up"() -> (w241:bool)
            n163 = Greater?(x=w249, y="Auto-Backup \nIdle Time (min)") -> (0:w244:bool)
            n164 = Greater?(x=w249, y="Auto-Standby\nTime (min)") -> (0:w236:bool)
            n165 = Not(x=w241) -> (.not. x?=w243:bool)
            n166 = case shown="True" w236 {
              tunnel: [FALSE ("Sleeping") w286] -> w245
              frame False {
              }
              frame True {
                w286 = TRUE
                n167 = property on="Sleep" class="Bool (strict)"("Val(Sgnl)"=w286) -> ()  [unwired: 2 in, 2 out]
              }
            }
            "Sleeping" <- w245
            n168 = And(x=w244, y=w243) -> (x .and. y?=w242:bool)
            n169 = case shown="False" w242 {
              frame False {
              }
              frame True {
                n170 = local read "SavePath"() -> (w287:path)
                n171 = String To IP() -> (0:w291:u32)  [unwired: 1 in]
                n172 = IP To String(2:w291) -> (0:w288:string)  [unwired: 1 in]
                n173 = Get Date/Time In Seconds() -> (seconds since 1Jan1904=w293:timestamp)
                n174 = Format Date/Time String(time format string (%c)="%Y-%m-%d-*", seconds (now)=w293) -> (date/time string=w290:string)  [unwired: 1 in]
                n175 = call "create unique folder.vi"("string"=w288, "path 2"=w287) -> ("path"=w296:path)  [unwired: 9 in]
                n176 = Concatenate Strings(w290, ".csv" ("string")) -> (w295:string)
                n177 = call <vilib>:"Recursive File List.vi"("pattern"=w295, "Folder Path"=w296) -> ("Number of Files"=w297:i32)  [unwired: 5 in, 4 out]
                n178 = Equal To 0?(x=w297) -> (x = 0?=w289:bool)
                n179 = case shown="True" w289 {
                  frame False {
                  }
                  frame True {
                    n180 = property on="Backup" class="Bool (strict)"("Val(Sgnl)"=TRUE) -> ()  [unwired: 2 in, 2 out]
                  }
                }
              }
            }
          }
          frame "Interpreter", Default {
            n181 = stacked-sequence {
              tunnel: w303 -> [_ w319 _ _ _]
              tunnel: w302 -> [w304 w318 _ w404 _]
              frame #0 {
                n182 = Index Array(array=w304, index (col)=0 ("disabled index (col)")) -> (element=w309:string[])  [unwired: 1 in]
                n183 = local read "Command Line"() -> (w308:string)
                n184 = Search 1D Array(1D array=w309, element=w308) -> (index of element=w307:i32)  [unwired: 1 in]
                n185 = Index Array(array=w304, index (row)=w307, index (col)=1 ("disabled index (col)")) -> (element=→"Laser Response":string)
              }
              frame #1 {
                n186 = for {
                  tunnel: w319 -> [w321] mode=indexing
                  tunnel: w318 -> [w322]
                  n187 = Index Array(array=w322, index (col)=0 ("disabled index (col)")) -> (element=w325:string[])  [unwired: 1 in]
                  n188 = Search 1D Array(1D array=w325, element=w321) -> (index of element=w323:i32)  [unwired: 1 in]
                  n189 = Index Array(array=w322, index (row)=w323, index (col)=1 ("disabled index (col)")) -> (element=w320:string)
                  n190 = case shown="\"?RH\"" w321 {
                    tunnel: w320 -> [_ w327 w329 w337 w338 w345 w354 w356 w364 w366 w368 w370 w371 w382 w384]
                    frame "False", Default {
                    }
                    frame "?L" {
                      n191 = Decimal String To Number(string=w327) -> (number=→"Laser Info":i32)  [unwired: 2 in, 1 out]
                    }
                    frame "?SHUTTER" {
                      n192 = Decimal String To Number(string=w329) -> (number=w330:i32)  [unwired: 2 in, 1 out]
                      n193 = local read "Shutter"() -> (w333:bool)
                      n194 = Not Equal To 0?(x=w330) -> (x != 0?=w332:bool)
                      n195 = And(x=w332, y=w333) -> (x .and. y?=w331:bool)
                      n196 = case shown="False" w331 {
                        frame False {
                          n197 = property on="Shutter" class="Bool (strict)"("Colors [4]"=cluster{u32, u32}[] [{12369084, 12369084}, {12369084, 12369084}]) -> ()  [unwired: 2 in, 2 out]
                        }
                        frame True {
                          n198 = property on="Shutter" class="Bool (strict)"("Colors [4]"=cluster{u32, u32}[] [{12369084, 12369084}, {6618880, 6618880}]) -> ()  [unwired: 2 in, 2 out]
                        }
                      }
                    }
                    frame "?VW" {
                      n199 = Decimal String To Number(string=w337) -> (number=w336:i32)  [unwired: 2 in, 1 out]
                      n200 = property on="Wavelength" class="DigNum (strict)"("Value"=w336) -> ()  [unwired: 2 in, 2 out]
                      n201 = shared-variable ".\\Laser Library.lvlib\\WV"(w336) -> ()  [unwired: 1 in, 1 out]
                    }
                    frame "?ALIGN" {
                      n202 = Decimal String To Number(string=w338) -> (number=w339:i32)  [unwired: 2 in, 1 out]
                      n203 = Not Equal To 0?(x=w339) -> (x != 0?=w342:bool)
                      n204 = local read "Align"() -> (w341:bool)
                      n205 = And(x=w342, y=w341) -> (x .and. y?=w340:bool)
                      n206 = case shown="False" w340 {
                        frame False {
                          n207 = property on="Align" class="Bool (strict)"("Colors [4]"=cluster{u32, u32}[] [{12369084, 12369084}, {12369084, 12369084}]) -> ()  [unwired: 2 in, 2 out]
                        }
                        frame True {
                          n208 = property on="Align" class="Bool (strict)"("Colors [4]"=cluster{u32, u32}[] [{12369084, 12369084}, {6618880, 6618880}]) -> ()  [unwired: 2 in, 2 out]
                        }
                      }
                    }
                    frame "?PHLDP" {
                      n209 = Decimal String To Number(string=w345) -> (number=w346:i32)  [unwired: 2 in, 1 out]
                      n210 = Not Equal To 0?(x=w346) -> (x != 0?=w349:bool)
                      n211 = local read "Dither hold"() -> (w347:bool)
                      n212 = And(x=w349, y=w347) -> (x .and. y?=w348:bool)
                      n213 = case shown="False" w348 {
                        frame False {
                          n214 = property on="Dither hold" class="Bool (strict)"("Colors [4]"=cluster{u32, u32}[] [{12369084, 12369084}, {12369084, 12369084}]) -> ()  [unwired: 2 in, 2 out]
                        }
                        frame True {
                          n215 = property on="Dither hold" class="Bool (strict)"("Colors [4]"=cluster{u32, u32}[] [{12369084, 12369084}, {6618880, 6618880}]) -> ()  [unwired: 2 in, 2 out]
                        }
                      }
                    }
                    frame "?UF" {
                      n216 = Decimal String To Number(string=w354) -> (number=w353:i32)  [unwired: 2 in, 1 out]
                      n217 = Round To Nearest(number=w353) -> (nearest integer value=→"Power (mW)":i32)
                    }
                    frame "?GDD" {
                      n218 = Decimal String To Number(string=w356) -> (number=w355:i32)  [unwired: 2 in, 1 out]
                      n219 = property on="GDD" class="DigNum (strict)"("Value"=w355) -> ()  [unwired: 2 in, 2 out]
                      n220 = shared-variable "My Computer\\Laser Library.lvlib\\GDD"(w355) -> ()  [unwired: 1 in, 1 out]
                    }
                    frame "?GDDMAX" {
                      n221 = Decimal String To Number(string=w364) -> (number=w362:i32)  [unwired: 2 in, 1 out]
                      n222 = Divide(x=w362, y=1000.0) -> (x/y=w358:dbl)
                      n223 = Round To Nearest(number=w358) -> (nearest integer value=w357:dbl)
                      n224 = Number To Decimal String(number=w357) -> (decimal integer string=w361:string)  [unwired: 1 in]
                      n225 = Concatenate Strings(w361, "k" ("string")) -> (→"Max":string)
                    }
                    frame "?TS" {
                      n226 = Decimal String To Number(string=w366) -> (number=→"Tunning Status":i32)  [unwired: 2 in, 1 out]
                    }
                    frame "?MDLK" {
                      n227 = Decimal String To Number(string=w368) -> (number=w369:i32)  [unwired: 2 in, 1 out]
                      n228 = Not Equal To 0?(x=w369) -> (x != 0?=→"ModeLocked":bool)
                    }
                    frame "?ST" {
                      "Operating Status" <- w370
                    }
                    frame "?F" {
                      "Faults" <- w371
                    }
                    frame "?RH" {
                      n229 = local read "Humidity Threshold"() -> (w372:dbl)
                      n230 = Decimal String To Number(string=w382) -> (number=w381:i32)  [unwired: 2 in, 1 out]
                      n231 = Greater?(x=w381, y=w372) -> (0:w380:bool)
                      n232 = local read "Operating Status"() -> (w375:string)
                      n233 = local read "Laser Info"() -> (w378:i32)
                      n234 = Select(t=2, s=w380, f=w378) -> (s? t:f=w379:i32)
                      n235 = Concatenate Strings(w375, "\nHigh Humidity") -> (w373:string)
                      n236 = Select(t=w373, s=w380, f=w375) -> (s? t:f=w376:string)
                      n237 = local write "Laser Info"(w379) -> ()
                      n238 = local write "Operating Status"(w376) -> ()
                    }
                    frame "?BT" {
                      n239 = Decimal String To Number(string=w384) -> (number=→"Baseplate Temp (C)":i32)  [unwired: 2 in, 1 out]
                    }
                  }
                }
                n240 = local read "Operating Status"() -> (w314:string)
                n241 = local read "Faults"() -> (w312:string)
                n242 = Decimal String To Number(string=w312) -> (number=w313:i32)  [unwired: 2 in, 1 out]
                n243 = Equal To 0?(x=w313) -> (x = 0?=w311:bool)
                n244 = Select(t=w314, s=w311, f=w312) -> (s? t:f=w315:string)
                n245 = Initialize Array(w315, 4 ("dimension size")) -> (w316:string[])
                n246 = property on="Laser Status" class="Bool (strict)"("Strings [4]"=w316) -> ()  [unwired: 2 in, 2 out]
              }
              frame #2 {
                n247 = local read "Tunning Status"() -> (w385:i32)
                n248 = local read "Laser Info"() -> (w389:i32)
                n249 = Equal To 0?(x=w385) -> (x = 0?=w386:bool)
                n250 = Equal?(x=0, y=w389) -> (x = y?=w387:bool)
                n251 = And(x=w386, y=w387) -> (x .and. y?=w388:bool)
                n252 = Equal?(x=w389, y=2.0) -> (x = y?=w392:bool)
                n253 = case shown="True" w392 {
                  tunnel: w388 -> [w393 _]
                  frame False {
                    n254 = case shown="False" w393 {
                      frame False {
                        w395 = TRUE ("Laser Status")
                        n255 = local read "Operating Status"() -> (w394:string)
                        n256 = local write "Laser Control"(w395) -> ()
                        n257 = local write "Laser Status"(w395) -> ()
                        n258 = Equal?(x=w394, y="OK") -> (x = y?=w396:bool)
                        n259 = case shown="False" w396 {
                          frame False {
                            n260 = property on="Laser Status" class="Bool (strict)"("Colors [4]"=cluster{u32, u32}[] [{16762130, 16762130}, {10441728, 10441728}, {10441728, 10441728}]) -> ()  [unwired: 2 in, 2 out]
                          }
                          frame True {
                            n261 = property on="Laser Status" class="Bool (strict)"("Colors [4]"=cluster{u32, u32}[] [{6618880, 6618880}]) -> ()  [unwired: 2 in, 2 out]
                          }
                        }
                      }
                      frame True {
                        w401 = FALSE
                        n262 = local write "Laser Control"(w401) -> ()
                        n263 = property on="Laser Status" class="Bool (strict)"("Colors [4]"=cluster{u32, u32}[] [{10682272, 10682272}, {12451729, 12451729}]) -> ()  [unwired: 2 in, 2 out]
                        "Laser Status" <- w401
                      }
                    }
                  }
                  frame True {
                    n264 = property on="Laser Status" class="Bool (strict)"("Colors [4]"=cluster{u32, u32}[] [{16723218, 15670016}, {16721170, 16725034}]) -> ()  [unwired: 2 in, 2 out]
                  }
                }
              }
              frame #3 {
                w406 = 2.0 ("y")
                w409 = 30
                n265 = Array Size(array=w404) -> (size(s)=w420:i32[])
                n266 = Index Array(array=w420, index=0) -> (element=w417:i32)
                n267 = Index Array(array=w420, index=1) -> (element=w416:i32)
                n268 = Multiply(x=w417, y=w416) -> (x*y=w414:i32)
                n269 = Divide(x=w414, y=w409) -> (x/y=w415:dbl)
                n270 = Divide(x=w409, y=w406) -> (x/y=w410:dbl)
                n271 = Reshape Array(w404, w414) -> (w413:string[])
                n272 = Subtract(x=w406, y=2.0) -> (x-y=w407:dbl)
                n273 = Round Toward +Infinity(x=w415) -> (ceil(x): smallest int >= x=w408:dbl)
                n274 = Initialize Array("", w410, w407) -> (w411:string[][])
                n275 = for {
                  N: w408 -> [_]
                  tunnel: w409 -> [w434]
                  shift-right: [w432] -> _
                  shift-left: w413 -> [w433]
                  tunnel: w409 -> [w428]
                  tunnel: w406 -> [w421]
                  shift-right: [w422] -> w403
                  shift-left: w411 -> [w424]
                  i -> [w431]
                  n276 = Divide(x=w428, y=w421) -> (x/y=w427:dbl)
                  n277 = Multiply(x=w431, y=w421) -> (x*y=w423:dbl)
                  n278 = Round Toward -Infinity(1:w427) -> (0:w426:dbl)
                  n279 = Split 1D Array(array=w433, index=w434) -> (first subarray=w430:string[], second subarray=w432:string[])
                  n280 = Reshape Array(w430, w426, 2 ("dimension size")) -> (w425:string[][])
                  n281 = Insert Into Array(array=w424, index (col)=w423, new element=w425) -> (w422:string[][])  [unwired: 1 in]
                }
                "Query List" <- w403
              }
              frame #4 {
                n282 = shared-variable ".\\Laser Library.lvlib\\Remote WV"() -> (w435:dbl)  [unwired: 1 in, 1 out]
                n283 = feedback-in #1(w435) -> ()
                n284 = feedback #1(w435) -> (w437:dbl)
                n285 = Not Equal?(x=w435, y=w437) -> (x != y?=w436:bool)
                n286 = case shown="True" w436 {
                  tunnel: w435 -> [_ w438]
                  frame False {
                  }
                  frame True {
                    n287 = property on="Wavelength" class="DigNum (strict)"("Val(Sgnl)"=w438) -> ()  [unwired: 2 in, 2 out]
                  }
                }
              }
            }
            n288 = local read "State next step"() -> (w301:string)
            "queue #" <- w300
          }
          frame "Walker" {
            w445 = dbl[] [680.0, 730.0, 780.0, 830.0, 880.0, 930.0, 980.0, 1030.0, 980.0, 930.0, 880.0, 830.0, 780.0, 730.0, 680.0, 800.0] ("Array")
            n289 = Wait (ms)(milliseconds to wait=2000) -> ()  [unwired: 1 out]
            n290 = local read "Step"() -> (w447:dbl)
            n291 = Index Array(array=w445, index=w447) -> (element=w441:dbl)
            n292 = Array Size(array=w445) -> (size(s)=w444:i32)
            n293 = Increment(x=w447) -> (x+1=w443:dbl)
            n294 = property on="Wavelength" class="DigNum (strict)"("Val(Sgnl)"=w441) -> ()  [unwired: 2 in, 2 out]
            n295 = Equal?(x=w443, y=w444) -> (x = y?=w442:bool)
            n296 = case shown="True" w442 {
              tunnel: w443 -> [w450 _]
              tunnel: [TRUE FALSE ("Walking")] -> w440
              frame False {
                n297 = local write "Step"(w450) -> ()
              }
              frame True {
                n298 = local write "WV Walk"(FALSE) -> ()
                n299 = local write "State next step"("Writer") -> ()
              }
            }
            "Walking" <- w440
          }
          frame "Backuper" {
            n300 = local read "Backuper state"() -> (w455:string)
            n301 = case shown="\"BackupFinal\"" w455 {
              tunnel: w457 -> [_ w480]
              frame "BackupInit", Default {
                n302 = flat-sequence {
                  frame #0 {
                    n303 = Wait (ms)(milliseconds to wait=u32 30000) -> ()  [unwired: 1 out]
                    n304 = local write "Backuper state"("BackupFinal") -> ()
                  }
                  frame #1 {
                    n305 = local write "Refresh"(TRUE ("Refresh")) -> ()
                  }
                }
              }
              frame "BackupFinal" {
                n306 = local write "Backup"(FALSE ("Backup")) -> ()
                n307 = local write "State next step"("Writer") -> ()
                n308 = local write "Backuper state"("BackupInit") -> ()
                n309 = local read "SavePath"() -> (w461:path)
                n310 = String To IP() -> (0:w474:u32)  [unwired: 1 in]
                n311 = IP To String(2:w474) -> (0:w462:string)  [unwired: 1 in]
                n312 = call "create unique folder.vi"("string"=w462, "path 2"=w461) -> ("path"=w467:path)  [unwired: 9 in]
                n313 = Get Date/Time In Seconds() -> (seconds since 1Jan1904=w476:timestamp)
                n314 = Format Date/Time String(time format string (%c)="%Y-%m-%d-%H-%M-%S", seconds (now)=w476) -> (date/time string=w471:string)  [unwired: 1 in]
                n315 = Path To String(path=w467) -> (string=w473:string)
                n316 = Concatenate Strings(w473, "\\" ("string"), w471, ".csv" ("string")) -> (w470:string)
                n317 = String To Path(string=w470) -> (path=w469:path)
                n318 = call-poly <vilib>:"Write To Spreadsheet File.vi"("delimiter (\\t)"="," ("delimiter (\\t)"), "format (%s)"="%.6f" ("format (%.3f)"), "append to file? (new file:F)"=FALSE, "2D data"=w480, "file path (dialog if empty)"=w469) -> ()  [unwired: 2 in, 2 out]
                "Backing up" <- FALSE ("Backing up ...")
              }
            }
          }
          frame "Quiter" {
            n319 = Equal To 0?(x=w485) -> (x = 0?=w484:bool)
            n320 = case shown="True" w484 {
              tunnel: ["Quiter" "Writer"] -> w483
              tunnel: [FALSE w489] -> w482
              frame False {
              }
              frame True {
                n321 = local read "Sleep"() -> (w488:bool)
                n322 = case shown="True" w488 {
                  tunnel: [w492 _] -> w489
                  frame False {
                    n323 = local read "QUIT"() -> (w491:bool)
                    n324 = case shown="True" w491 {
                      tunnel: [_ w493] -> w492
                      frame False {
                      }
                      frame True {
                        w493 = TRUE
                        n325 = local write "QUIT"(FALSE) -> ()
                        n326 = local write "stop"(w493) -> ()
                      }
                    }
                  }
                  frame True {
                    w495 = FALSE ("Sleep")
                    n327 = property on="Laser Control" class="Bool (strict)"("Val(Sgnl)"=w495) -> ()  [unwired: 2 in, 2 out]
                    n328 = local write "Sleeping"(w495) -> ()
                    n329 = local write "Sleep"(w495) -> ()
                    n330 = local write "State next step"("Writer" ("State next step")) -> ()
                  }
                }
              }
            }
          }
        }
      }
      n331 = VISA Close(VISA resource name=w59, error in (no error)=w58) -> (error out=w64:errorcluster)
      n332 = call <vilib>:"Simple Error Handler.vi"("error in (no error)"=w64) -> ()  [unwired: 1 in, 8 out]
    }
  }
